vi "CalculatedValues.vi"(8 "CCM LM":dbl[][](array[numeric]), 9 "CCM H":dbl[][](array[numeric]), 10 "Calculated Values":T1, 11 "Data":T2 caption="All Data Cluster") -> (3 "Calculated Values":T1)   [LabVIEW 2018, in "Controller (Host).lvlib"]
uses:
  Controller (Host).lvlib
  Top Level/Shared Controls/Calculated Data.ctl
  Top Level/Shared Controls/All Data Cluster.ctl
  Top Level/Shared Controls/Acq Data.ctl
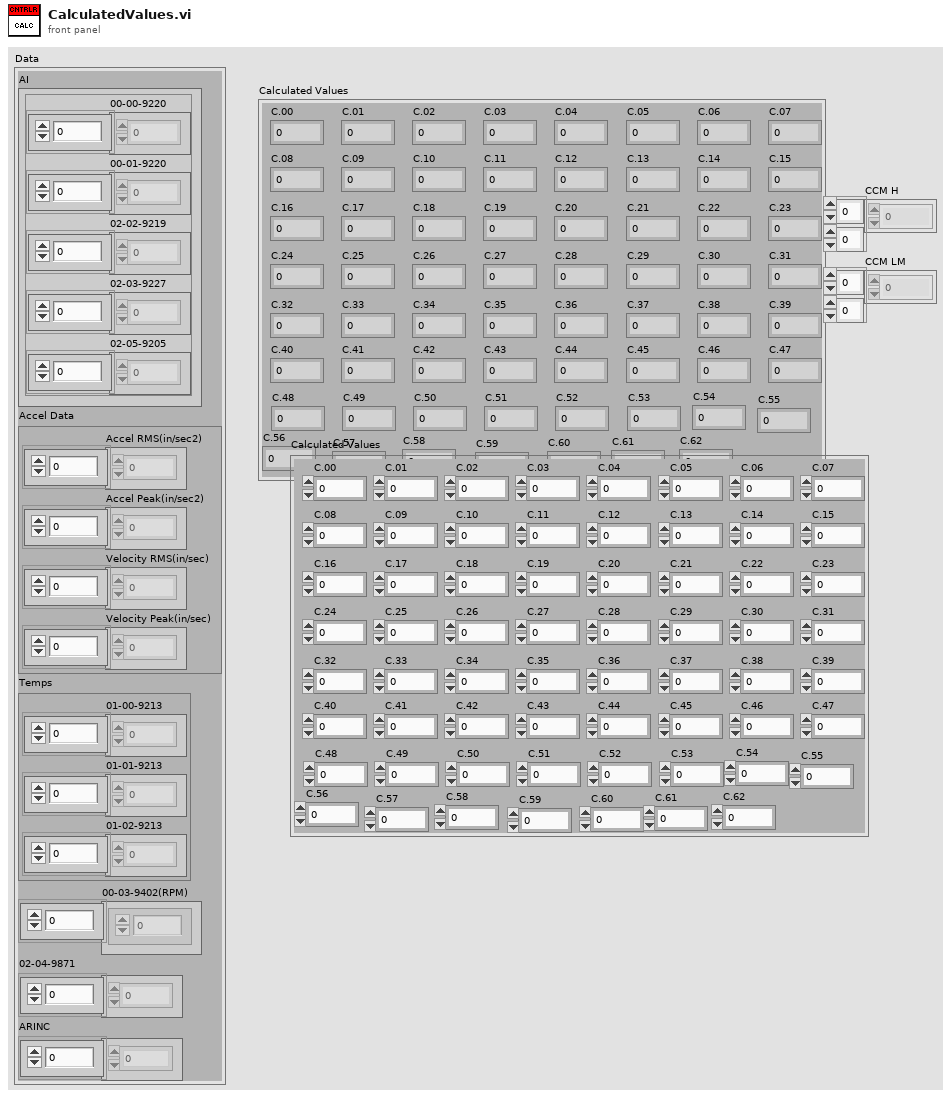
[diagram p1: front panel]
types:
  T1 = typedef "Calculated Data.ctl" = cluster{"C.00":dbl, "C.01":dbl, "C.02":dbl, "C.03":dbl, "C.04":dbl, "C.05":dbl, "C.06":dbl, "C.07":dbl, "C.08":dbl, "C.09":dbl, "C.10":dbl, "C.11":dbl, "C.12":dbl, "C.13":dbl, "C.14":dbl, "C.15":dbl, "C.16":dbl, "C.17":dbl, "C.18":dbl, "C.19":dbl, "C.20":dbl, "C.21":dbl, "C.22":dbl, "C.23":dbl, "C.24":dbl, "C.25":dbl, "C.26":dbl, "C.27":dbl, "C.28":dbl, "C.29":dbl, "C.30":dbl, "C.31":dbl, "C.32":dbl, "C.33":dbl, "C.34":dbl, "C.35":dbl, "C.36":dbl, "C.37":dbl, "C.38":dbl, "C.39":dbl, "C.40":dbl, "C.41":dbl, "C.42":dbl, "C.43":dbl, "C.44":dbl, "C.45":dbl, "C.46":dbl, "C.47":dbl, "C.48":dbl, "C.49":dbl, "C.50":dbl, "C.51":dbl, "C.52":dbl, "C.53":dbl, "C.54":dbl, "C.55":dbl, "C.56":dbl, "C.57":dbl, "C.58":dbl, "C.59":dbl, "C.60":dbl, "C.61":dbl, "C.62":dbl}
  T2 = typedef "All Data Cluster.ctl" = cluster{"AI":T3, "Accel Data":cluster{"Accel RMS(in/sec2)":dbl[], "Accel Peak(in/sec2)":dbl[], "Velocity RMS(in/sec)":dbl[], "Velocity Peak(in/sec)":dbl[]}, "Temps":cluster{"01-00-9213":dbl[], "01-01-9213":dbl[], "01-02-9213":dbl[]}, "00-03-9402(RPM)":dbl[], "02-04-9871":dbl[], "ARINC":sgl[]}
  T3 = typedef "Acq Data.ctl" = cluster{"00-00-9220":dbl[], "00-01-9220":dbl[], "02-02-9219":dbl[], "02-03-9227":dbl[], "02-05-9205":dbl[]}
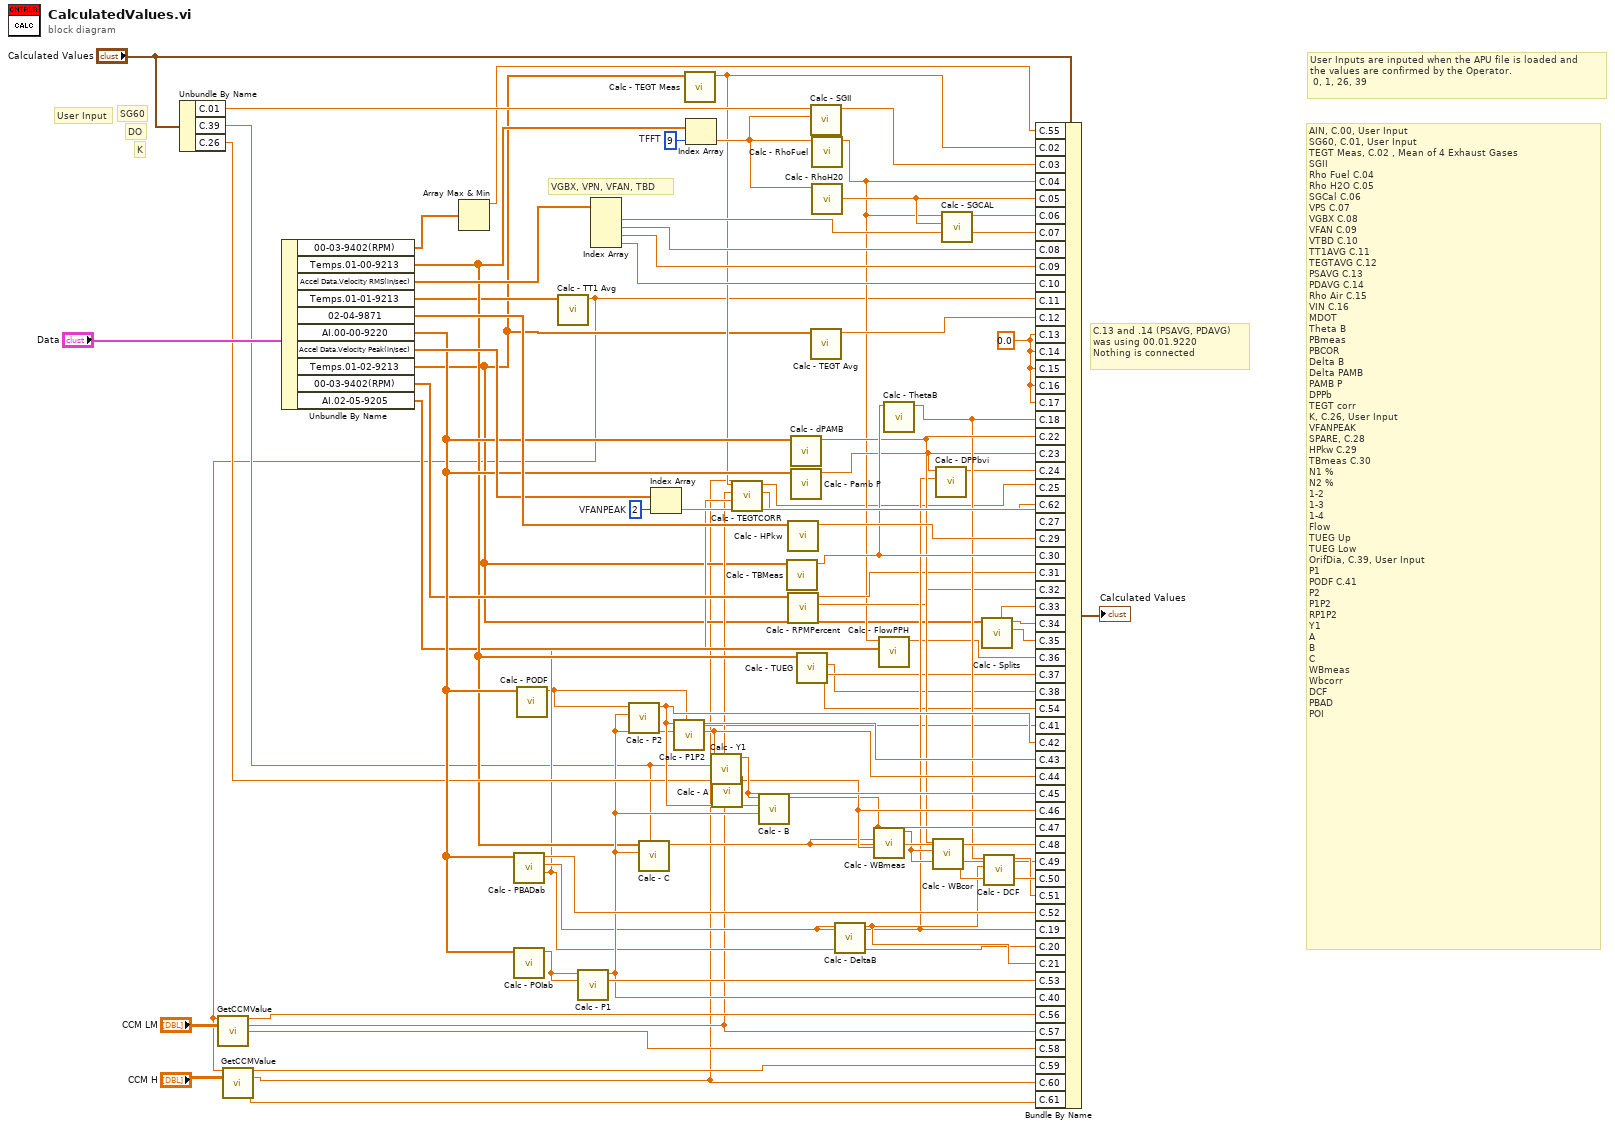
[diagram p0: block diagram]
diagram:
  w10 = 0.0 ("C.13")
  w57 = 2  # VFANPEAK
  w71 = 9  # TFFT
  # "K"
  # "DO"
  # "SG60"
  # "User Input"
  # "VGBX, VPN, VFAN, TBD"
  # "C.13 and .14 (PSAVG, PDAVG)\nwas using 00.01.9220\nNothing is connected"
  # "User Inputs are inputed when the APU file is loaded and \nthe values are confirmed by the Operator. \n 0, 1, 26, 39"
  # "AIN, C.00, User Input\nSG60, C.01, User Input\nTEGT Meas, C.02 , Mean of 4 Exhaust Gases\nSGII\nRho Fuel C.04\nRho H2O C.05\nSGCal C.06\nVPS C.07\nVGBX C.08\nVFAN C.09\nVTBD C.10\nTT1AVG C.11\nTEGTAVG C.12\nPSAVG C.13\nPDAVG C.14\nRho Air C.15\nVIN C.16\nMDOT\nTheta B\nPBmeas\nPBCOR\nDelta B\nDelta PAMB\nPAMB P\nDPPb\nTEGT corr\nK, C.26, User Input\nVFANPEAK\nSPARE, C.28\nHPkw C.29\nTBmeas C.30\nN1 %\nN2 %\n1-2\n1-3\n1-4\nFlow\nTUEG Up\nTUEG Low\nOrifDia, C.39, User Input\nP1\nPODF C.41\nP2\nP1P2\nRP1P2\nY1\nA\nB\nC\nWBmeas\nWbcorr\nDCF\nPBAD\nPOI"
  n1 = Unbundle By Name("Calculated Values") -> ("C.01"=w62:dbl, "C.39"=w8:dbl, "C.26"=w47:dbl)
  n2 = Unbundle By Name("Data") -> ("00-03-9402(RPM)"=w17:dbl[], "Temps.01-00-9213"=w27:dbl[], "Accel Data.Velocity RMS(in/sec)"=w67:dbl[], "Temps.01-01-9213"=w12:dbl[], "02-04-9871"=w59:dbl[], "AI.00-00-9220"=w54:dbl[], "Accel Data.Velocity Peak(in/sec)"=w58:dbl[], "Temps.01-02-9213"=w11:dbl[], "00-03-9402(RPM)"=w33:dbl[], "AI.02-05-9205"=w23:dbl[])
  n3 = Array Max & Min(array=w17) -> (max value=w16:dbl)  [unwired: 3 out]
  n4 = call "Calc - PBADab.vi"("00-00-9220"=w54) -> ("PBCOR"=w20:dbl, "PBMeasP"=w36:dbl, "PBADab"=w55:dbl)  [unwired: 8 in]
  n5 = call "Calc - POIab.vi"("00-00-9220"=w54) -> ("POIab"=w53:dbl)  [unwired: 10 in]
  n6 = call "Calc - PODF.vi"("00-00-9220"=w54) -> ("PODF"=w9:dbl)  [unwired: 10 in]
  n7 = call "Calc - TT1 Avg.vi"("01-01-9213"=w12) -> ("TT1 Avg"=w5:dbl)  [unwired: 10 in]
  n8 = call "GetCCMValue.vi"("TT1 F"=w5, "CMM"="CCM LM") -> ("WBLimit"=w15:dbl, "PBLimit"=w14:dbl, "EGTLimit"=w13:dbl)  [unwired: 11 in]
  n9 = call "GetCCMValue.vi"("TT1 F"=w5, "CMM"="CCM H") -> ("WBLimit"=w4:dbl, "PBLimit"=w1:dbl, "EGTLimit"=w3:dbl)  [unwired: 11 in]
  n10 = call "Calc - P1.vi"("POIab"=w53) -> ("P1"=w46:dbl)  [unwired: 10 in]
  n11 = Index Array(array=w67) -> (element #1=w66:dbl, element #2=w65:dbl, element #3=w64:dbl, element #4=w63:dbl)  [unwired: 4 in]
  n12 = call "Calc - P2.vi"("P1"=w46, "PODF"=w9) -> ("P2"=w48:dbl)  [unwired: 9 in]
  n13 = call "Calc - C.vi"("DO"=w8, "P1"=w46, "Temps.01-00-9213"=w27) -> ("C"=w43:dbl)  [unwired: 8 in]
  n14 = Index Array(array=w58, index=w57) -> (element=w56:dbl)
  n15 = call "Calc - P1P2.vi"("P1"=w46, "P2"=w48) -> ("RP1P2"=w51:dbl, "P1P2"=w52:dbl)  [unwired: 8 in]
  n16 = call "Calc - TEGT Meas.vi"("01-02-9213"=w11) -> ("TEGT Meas"=w19:dbl)  [unwired: 10 in]
  n17 = Index Array(array=w27, index=w71) -> (element=w70:dbl)
  n18 = call "Calc - Y1.vi"("C.39"=w8, "RP1P2"=w51) -> ("Y1"=w49:dbl)  [unwired: 9 in]
  n19 = call "Calc - A.vi"("K"=w47) -> ("A"=w45:dbl)  [unwired: 10 in]
  n20 = call "Calc - TEGTCORR.vi"("PBLimitH"=w1, "PBCOR"=w20, "PBLimitLM"=w14, "TEGT Meas"=w19) -> ("TEGTCORRH"=w2:dbl, "TEGTCORRLM"=w21:dbl)  [unwired: 6 in]
  n21 = call "Calc - B.vi"("P1"=w46, "P2"=w48, "Y1"=w49) -> ("B"=w44:dbl)  [unwired: 8 in]
  n22 = call "Calc - TBMeas.vi"("01-02-9213"=w11) -> ("TBMeas"=w50:dbl)  [unwired: 10 in]
  n23 = call "Calc - HPkw.vi"("02-04-9871(Modbus)"=w59) -> ("HPKW"=w60:dbl)  [unwired: 10 in]
  n24 = call "Calc - RPMPercent.vi"("00-03-9402(RPM)"=w33) -> ("N2%"=w31:dbl, "N1%"=w32:dbl)  [unwired: 9 in]
  n25 = call "Calc - dPAMB.vi"("00-00-9220"=w54) -> ("dPAMB"=w42:dbl)  [unwired: 10 in]
  n26 = call "Calc - Pamb P.vi"("00-00-9220"=w54) -> ("Pamb P"=w35:dbl)  [unwired: 10 in]
  n27 = call "Calc - TUEG.vi"("01-00-9213"=w27) -> ("TUEGDelta"=w18:dbl, "TUEGLower"=w25:dbl, "TUEGUpper"=w26:dbl)  [unwired: 8 in]
  n28 = call "Calc - SGII.vi"("TFFT"=w70, "SG60"=w62) -> ("SG11"=w72:dbl)  [unwired: 9 in]
  n29 = call "Calc - TEGT Avg.vi"("01-02-9213"=w11) -> ("TEGT Avg"=w61:dbl)  [unwired: 10 in]
  n30 = call "Calc - RhoFuel.vi"("TFFT"=w70) -> ("RhoFuel"=w22:dbl)  [unwired: 10 in]
  n31 = call "Calc - RhoH20.vi"("TFFT"=w70) -> ("RhoH20"=w69:dbl)  [unwired: 10 in]
  n32 = call "Calc - DeltaB.vi"("PBMeas P"=w36) -> ("Delta B"=w37:dbl)  [unwired: 10 in]
  n33 = call "Calc - WBmeas.vi"("A"=w45, "C"=w43, "B"=w44) -> ("WBMeas"=w39:dbl)  [unwired: 8 in]
  n34 = call "Calc - FlowPPH.vi"("02-05-9205"=w23, "RhoFuel"=w22) -> ("FlowPPH"=w24:dbl)  [unwired: 9 in]
  n35 = call "Calc - ThetaB.vi"("TBMeas"=w50) -> ("ThetaB"=w38:dbl)  [unwired: 10 in]
  n36 = call "Calc - WBcor.vi"("WBMeas"=w39, "dPAMB"=w42) -> ("WBCor"=w41:dbl)  [unwired: 9 in]
  n37 = call "Calc - DPPbvi.vi"("PBMeas P"=w36, "PBAR"=w35) -> ("DPPb"=w34:dbl)  [unwired: 9 in]
  n38 = call "Calc - SGCAL.vi"("RhoH20"=w69, "RhoFuel"=w22) -> ("SGCAL"=w68:dbl)  [unwired: 9 in]
  n39 = call "Calc - Splits.vi"("01-02-9213"=w11) -> ("C.35"=w28:dbl, "C.34"=w29:dbl, "C.33"=w30:dbl)  [unwired: 8 in]
  n40 = call "Calc - DCF.vi"("WBMeas"=w39, "DeltaB"=w37, "ThetaB"=w38) -> ("DCF"=w40:dbl)  [unwired: 8 in]
  n41 = Bundle By Name(cluster="Calculated Values", "C.55"=w16, "C.02"=w19, "C.03"=w72, "C.04"=w22, "C.05"=w69, "C.06"=w68, "C.07"=w66, "C.08"=w65, "C.09"=w64, "C.10"=w63, "C.11"=w5, "C.12"=w61, "C.13"=w10, "C.14"=w10, "C.15"=w10, "C.16"=w10, "C.17"=w10, "C.18"=w38, "C.22"=w42, "C.23"=w35, "C.24"=w34, "C.25"=w21, "C.62"=w2, "C.27"=w56, "C.29"=w60, "C.30"=w50, "C.31"=w32, "C.32"=w31, "C.33"=w30, "C.34"=w29, "C.35"=w28, "C.36"=w24, "C.37"=w26, "C.38"=w25, "C.54"=w18, "C.41"=w9, "C.42"=w48, "C.43"=w52, "C.44"=w51, "C.45"=w49, "C.46"=w45, "C.47"=w44, "C.48"=w43, "C.49"=w39, "C.50"=w41, "C.51"=w40, "C.52"=w55, "C.19"=w36, "C.20"=w20, "C.21"=w37, "C.53"=w53, "C.40"=w46, "C.56"=w15, "C.57"=w14, "C.58"=w13, "C.59"=w4, "C.60"=w1, "C.61"=w3) -> (→"Calculated Values":T1)
